vi "Database Server Driver.vi"(4 "Create Table":T4={"table"="", "column information"=[], "primary key (-1)"=-1, "use file? (F)"=FALSE}, 5 "Insert Data":T1, 6 "Options":T6=enum."Select Data", 7 "SQLTableData":T5, 8 "error in":errorcluster, 9 "SQL query":string, 10 "Select":enum16{"SelectWithQuery", "SelectWithColumn"}(ring), 11 "table":string) -> (0 "error out":errorcluster, 1 "tables":string[](array[string]), 2 "Database out":refnum<class "Database.lvclass">, 3 "data":string[][](array[string]))   [LabVIEW 2023, in "HardwareAbstractionLayer_LVOOP.lvlib" / "Database.lvclass"]
doc: "This VI used to Database action engine.\n\n// Defeault Case Select Query"
uses:
  Database.lvclass
  Control/DB Options.ctl
  <vilib>/addons/database/Auxilliary.llb/DB Tools Column Info.ctl
  <vilib>/addons/database/Auxilliary.llb/DB Tools DataTypes.ctl
  MYSQL Database_class/MYSQL Database.lvclass
  SQLite Database_class/SQLite Database.lvclass
  Control/DB Selection.ctl
  MYSQL Server_class/MYSQL Server.lvclass
  <vilib>/addons/database/NI_Database_API.lvlib
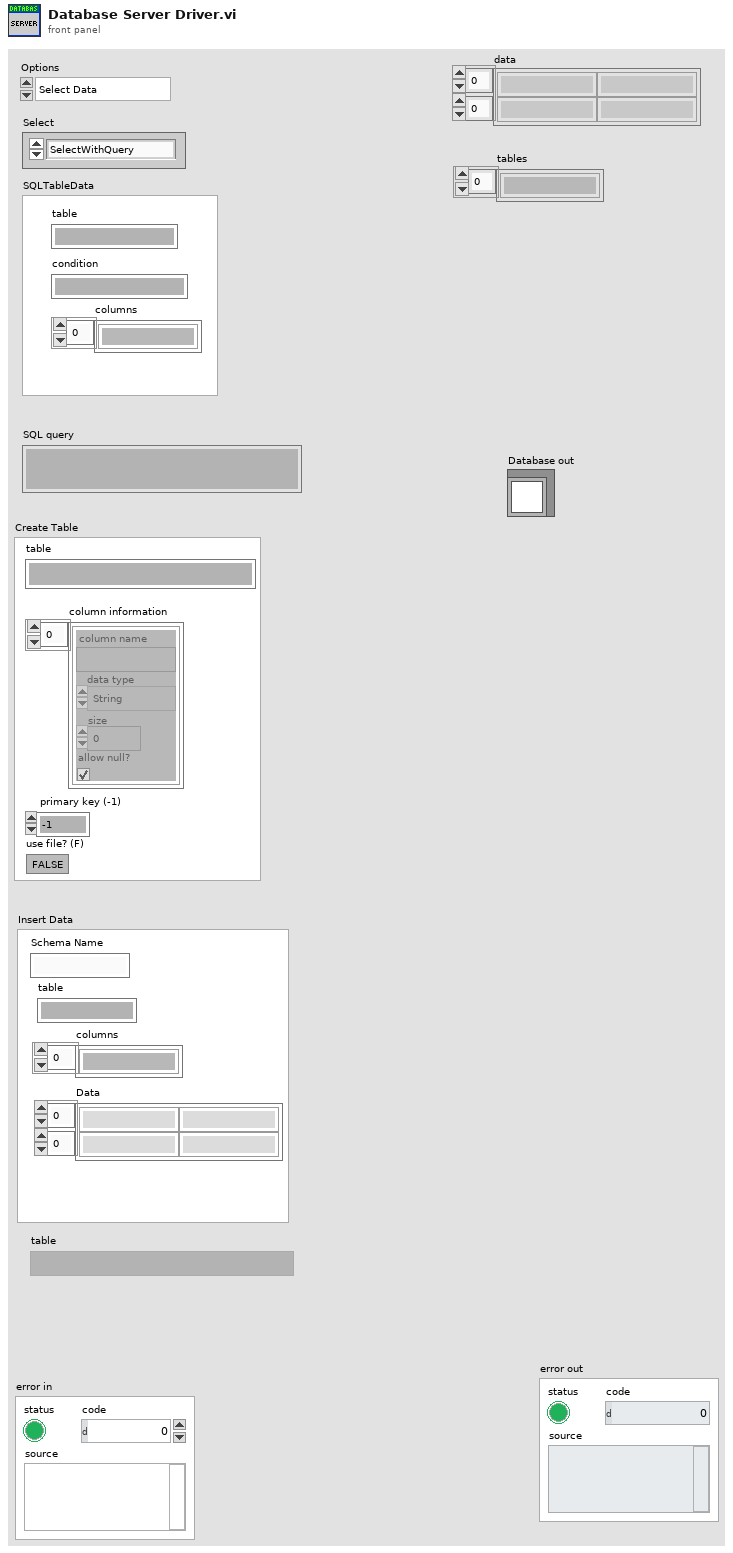
[diagram p1: front panel]
types:
  T1 = cluster{"table":string, "columns":string[], "Data":string[][], "Schema Name":string}
  T2 = typedef "NI_Database_API.lvlib/DB Tools Column Info.ctl" = cluster{"column name":string, "data type":T3, "size":i32, "allow null?":bool}
  T3 = typedef "NI_Database_API.lvlib/DB Tools DataTypes.ctl" = enum16{"String", "Long (I32)", "Single (SGL)", "Double (DBL)", "Date/Time", "Binary"}
  T4 = cluster{"table":string, "column information":T2[], "primary key (-1)":i32, "use file? (F)":bool}
  T5 = cluster{"table":string, "condition":string, "columns":string[]}
  T6 = typedef "HardwareAbstractionLayer_LVOOP.lvlib/Database.lvclass/DB Options.ctl" = enum16{"Init", "Select Data", "Insert Data", "Update Data", "Delete Data", "Execute Query", "Create Schema", "Create Table", "List Tables", "List Columns", "Close"}
  T7 = cluster{"DataSource Name":string, "userID":string, "password":string}
  T8 = enum16{"open", "replace", "create", "open or create", "replace or create", "replace or create with confirmation"}
  T9 = typedef "HardwareAbstractionLayer_LVOOP.lvlib/Database.lvclass/DB Selection.ctl" = string
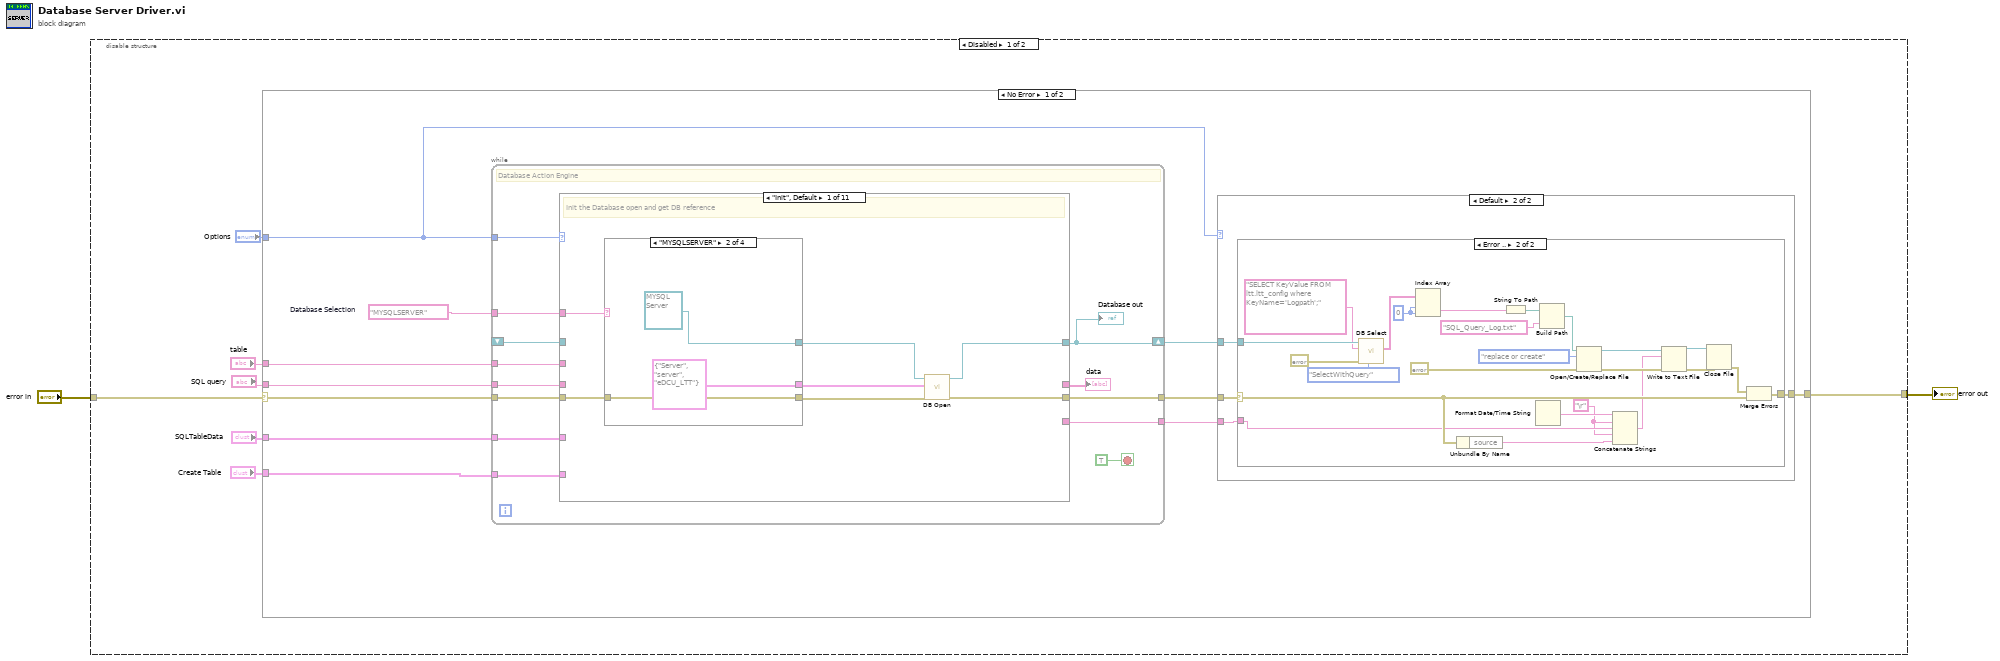
[diagram p0: block diagram]
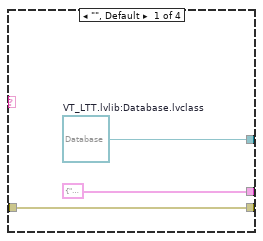
[diagram p2: hidden frame]
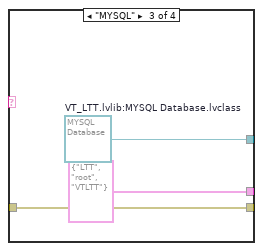
[diagram p3: hidden frame]
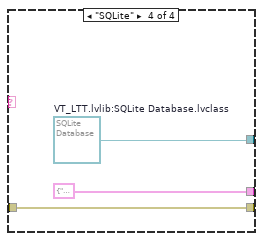
[diagram p4: hidden frame]
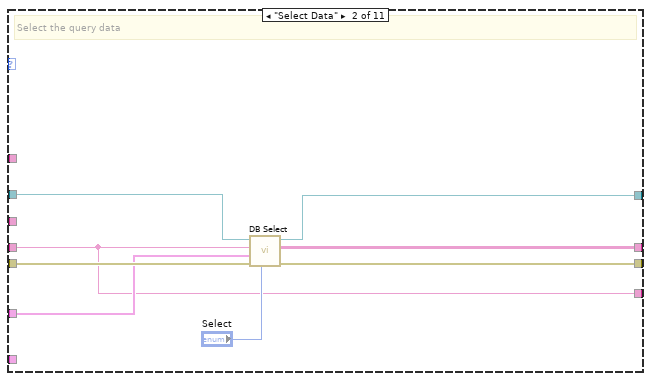
[diagram p5: hidden frame]
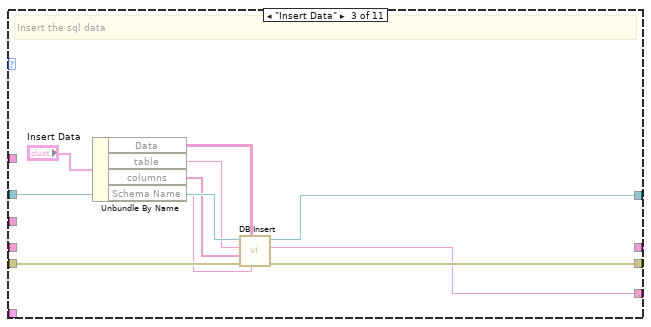
[diagram p6: hidden frame]
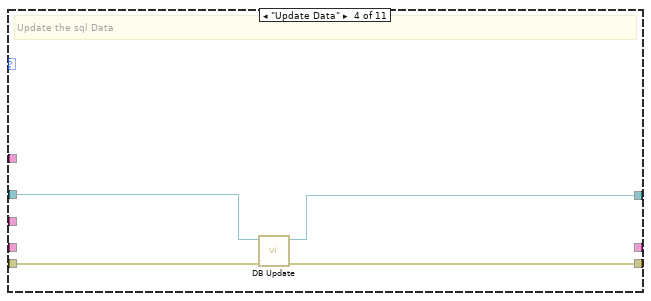
[diagram p7: hidden frame]
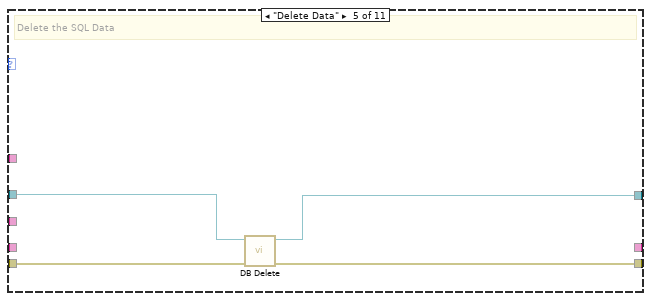
[diagram p8: hidden frame]
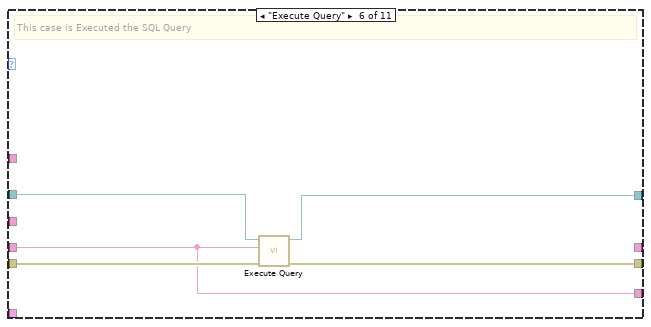
[diagram p9: hidden frame]
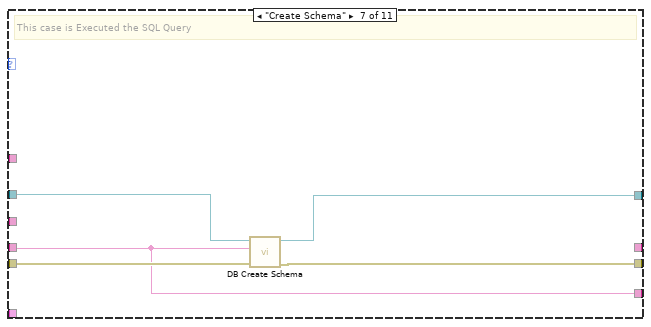
[diagram p10: hidden frame]
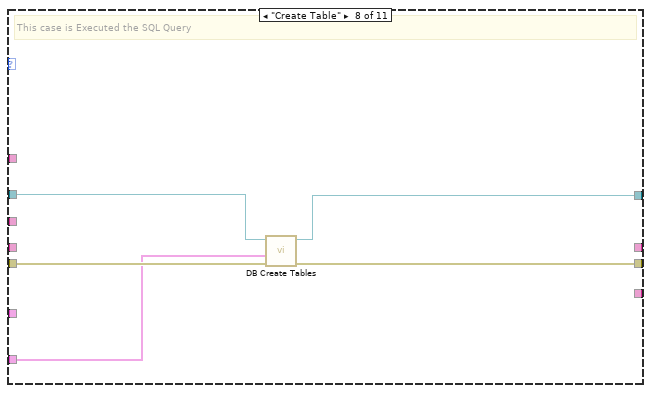
[diagram p11: hidden frame]
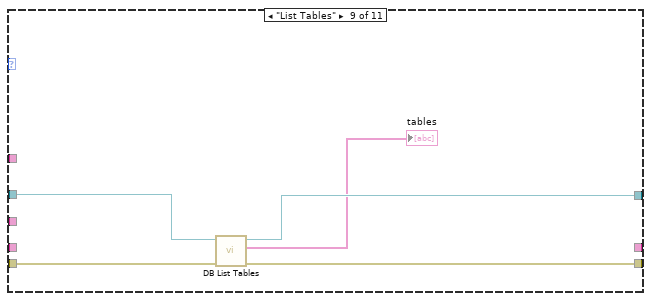
[diagram p12: hidden frame]
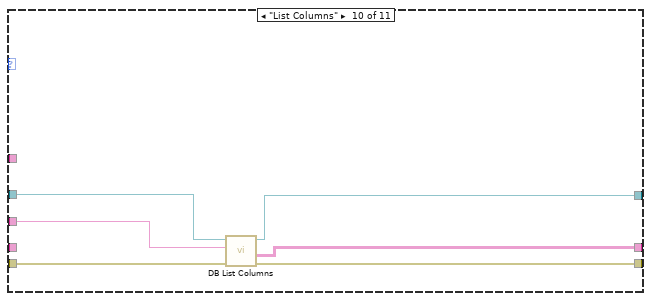
[diagram p13: hidden frame]
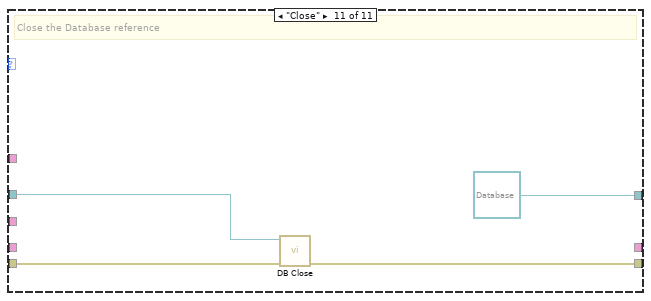
[diagram p14: hidden frame]
diagram:
  n1 = disable-structure shown="Disabled" {
    disable-tunnel: [w4 w140] -> w2
    disable-tunnel: "error in" -> [w3 w140]
    frame Disabled {
      n2 = case shown="No Error" w3 {
        selector: w3 -> [w19 w139]
        tunnel: "SQL query" -> [w18 _]
        tunnel: "SQLTableData" -> [w17 _]
        tunnel: "Create Table" -> [w16 _]
        tunnel: "table" -> [w15 _]
        tunnel: [w12 w139] -> w4
        tunnel: "Options" -> [w11 _]
        frame No Error {
          w20 = T9 "MYSQLSERVER"  # Database Selection
          n3 = while {
            tunnel: w11 -> [w32]
            tunnel: w20 -> [w31]
            shift-right: [w23] -> w10
            shift-left: _ -> [w28]
            tunnel: w18 -> [w27]
            tunnel: w17 -> [w26]
            tunnel: w16 -> [w24]
            tunnel: w15 -> [w22]
            tunnel: [w21] -> w13
            tunnel: w19 -> [w30]
            tunnel: [w29] -> w14
            stop <- TRUE stop-if-true
            # "Database Action Engine"
            n4 = case shown="\"Init\", Default" w32 {
              tunnel: w31 -> [w40 _ _ _ _ _ _ _ _ _ _]
              tunnel: w30 -> [w39 w60 w69 w74 w78 w83 w87 w91 w97 w103 w108]
              tunnel: [w34 w59 w68 w73 w77 w82 w86 w90 w96 w101 w107] -> w29
              tunnel: [w35 w57 w67 w71 w75 w80 w85 w92 w95 w102 refnum<class "Database.lvclass"> refnum ("Database out")] -> w23
              tunnel: w28 -> [_ w58 w70 w72 w76 w81 w88 w93 w98 w104 w106]
              tunnel: w27 -> [_ w53 _ _ _ w79 w84 _ _ _ _]
              tunnel: w26 -> [_ w55 _ _ _ _ _ _ _ _ _]
              tunnel: [_ w54 _ _ _ _ _ _ _ w99 _] -> w25
              tunnel: w24 -> [_ _ _ _ _ _ _ w89 _ _ _]
              tunnel: w22 -> [_ _ _ _ _ _ _ _ _ w100 _]
              tunnel: [_ w53 w61 _ _ w79 w84 _ _ _ _] -> w21
              frame "Init", Default {
                # "Init the Database open and get DB reference"
                n5 = case shown="\"MYSQLSERVER\"" w40 {
                  tunnel: w39 -> [w43 w46 w49 w52]
                  tunnel: [w43 w46 w49 w52] -> w38
                  tunnel: [w42 refnum<class "MYSQL Server.lvclass"> refnum ("HardwareAbstractionLayer_LVOOP.lvlib:MYSQL Server.lvclass") w48 w51] -> w37
                  tunnel: [T7 {"DataSource Name"="", "userID"="", "password"=""} ("DB") T7 {"DataSource Name"="Server", "userID"="server", "password"="eDCU_LTT"} ("DB") T7 {"DataSource Name"="LTT", "userID"="root", "password"="VTLTT"} ("DB") T7 {"DataSource Name"="", "userID"="", "password"=""} ("DB")] -> w36
                  frame "", Default {
                    w42 = refnum<class "Database.lvclass"> refnum  # VT_LTT.lvlib:Database.lvclass
                  }
                  frame "MYSQLSERVER" {
                  }
                  frame "MYSQL" {
                    w48 = refnum<class "MYSQL Database.lvclass"> refnum  # VT_LTT.lvlib:MYSQL Database.lvclass
                  }
                  frame "SQLite" {
                    w51 = refnum<class "SQLite Database.lvclass"> refnum  # VT_LTT.lvlib:SQLite Database.lvclass
                  }
                }
                n6 = call-dynamic "DB Open.vi"("error in"=w38, "DB"=w36, "Database in"=w37) -> ("error out"=w34:errorcluster, "Database out"=w35:refnum<class "Database.lvclass">)  [unwired: 7 in]
              }
              frame "Select Data" {
                # "Select the query data"
                n7 = call-dynamic "DB Select.vi"("Select"="Select", "error in (no error)"=w60, "SQLTableData"=w55, "SQL query"=w53, "Database in"=w58) -> ("error out"=w59:errorcluster, "data"=w54:string[][], "Database out"=w57:refnum<class "Database.lvclass">)  [unwired: 4 in]
              }
              frame "Insert Data" {
                # "Insert the sql data"
                n8 = Unbundle By Name("Insert Data") -> ("Data"=w63:string[][], "table"=w65:string, "columns"=w64:string[], "Schema Name"=w62:string)
                n9 = call-dynamic "DB Insert.vi"("Schema Name"=w62, "Data"=w63, "error in (no error)"=w69, "columns"=w64, "table"=w65, "Database in"=w70) -> ("error out"=w68:errorcluster, "SQL"=w61:string, "Database out"=w67:refnum<class "Database.lvclass">)  [unwired: 3 in]
              }
              frame "Update Data" {
                # "Update the sql Data"
                n10 = call-dynamic "DB Update.vi"("error in (no error)"=w74, "Database in"=w72) -> ("error out"=w73:errorcluster, "Database out"=w71:refnum<class "Database.lvclass">)  [unwired: 8 in]
              }
              frame "Delete Data" {
                # "Delete the SQL Data"
                n11 = call-dynamic "DB Delete.vi"("error in (no error)"=w78, "Database in"=w76) -> ("error out"=w77:errorcluster, "Database out"=w75:refnum<class "Database.lvclass">)  [unwired: 8 in]
              }
              frame "Execute Query" {
                # "This case is Executed the SQL Query"
                n12 = call-dynamic "Execute Query.vi"("error in (no error)"=w83, "SQL query"=w79, "Database in"=w81) -> ("error out"=w82:errorcluster, "Database out"=w80:refnum<class "Database.lvclass">)  [unwired: 7 in]
              }
              frame "Create Schema" {
                # "This case is Executed the SQL Query"
                n13 = call-dynamic "DB Create Schema.vi"("error in (no error)"=w87, "SQL query"=w84, "Database in"=w88) -> ("error out"=w86:errorcluster, "Database out"=w85:refnum<class "Database.lvclass">)  [unwired: 7 in]
              }
              frame "Create Table" {
                # "This case is Executed the SQL Query"
                n14 = call-dynamic "DB Create Tables.vi"("error in (no error)"=w91, "Create Table"=w89, "Database in"=w93) -> ("error out"=w90:errorcluster, "Database out"=w92:refnum<class "Database.lvclass">)  [unwired: 7 in]
              }
              frame "List Tables" {
                n15 = call-dynamic "DB List Tables.vi"("error in (no error)"=w97, "Database in"=w98) -> ("error out"=w96:errorcluster, "tables"=→"tables":string[], "Database out"=w95:refnum<class "Database.lvclass">)  [unwired: 7 in]
              }
              frame "List Columns" {
                n16 = call-dynamic "DB List Columns.vi"("error in (no error)"=w103, "table"=w100, "Database in"=w104) -> ("error out"=w101:errorcluster, "tableDetails"=w99:string[][], "Database out"=w102:refnum<class "Database.lvclass">)  [unwired: 5 in, 1 out]
              }
              frame "Close" {
                # "Close the Database reference"
                n17 = call-dynamic "DB Close.vi"("error in"=w108, "Database in"=w106) -> ("error out"=w107:errorcluster)  [unwired: 8 in, 1 out]
              }
            }
            "data" <- w25
            "Database out" <- w23
          }
          n18 = case shown="Default" w11 {
            tunnel: w14 -> [w109 w113]
            tunnel: w13 -> [_ w112]
            tunnel: [w109 w111] -> w12
            tunnel: w10 -> [_ w110]
            frame "Init", "Close" {
            }
            frame Default {
              n19 = case shown="Error .." w113 {
                selector: w113 -> [w114 w120]
                tunnel: w112 -> [_ w117]
                tunnel: [w114 w130] -> w111
                tunnel: w110 -> [_ w129]
                frame No Error {
                }
                frame Error {
                  w116 = "\r"
                  w125 = 0 ("disabled index (col)")
                  n20 = call-dynamic "DB Select.vi"("Select"=enum16{"SelectWithQuery", "SelectWithColumn"}."SelectWithQuery", "error in (no error)"=errorcluster {"status"=FALSE, "code"=0, "source"=""}, "SQL query"="SELECT KeyValue FROM ltt.ltt_config where KeyName='Logpath';", "Database in"=w129) -> ("data"=w126:string[][])  [unwired: 5 in, 2 out]
                  n21 = Index Array(array=w126, index (row)=w125, index (col)=w125) -> (element=w124:string)
                  n22 = Unbundle By Name(w120) -> ("source"=w115:string)
                  n23 = String To Path(string=w124) -> (path=w123:path)
                  n24 = Format Date/Time String() -> (date/time string=w119:string)  [unwired: 3 in]
                  n25 = Build Path(base path=w123, name or relative path="SQL_Query_Log.txt") -> (appended path=w132:path)
                  n26 = Open/Create/Replace File(file path (use dialog)=w132, error in=errorcluster {"status"=FALSE, "code"=0, "source"=""}, operation (0:open)=T8."replace or create") -> (refnum out=w136:refnum<file>, error out=w135:errorcluster)  [unwired: 3 in, 1 out]
                  n27 = Concatenate Strings(w119, w116, w117, w116, w115) -> (w118:string)
                  n28 = Write to Text File(file (use dialog)=w136, text=w118, error in=w135) -> (refnum out=w138:refnum<file>, error out=w137:errorcluster)  [unwired: 1 in, 1 out]
                  n29 = Close File(refnum=w138, error in=w137) -> (error out=w131:errorcluster)  [unwired: 1 out]
                  n30 = Merge Errors(w131, w120) -> (w130:errorcluster)
                }
              }
            }
          }
        }
        frame Error {
        }
      }
    }
    frame Enabled {
    }
  }
  "error out" <- w2
